vi "destroySubDataUserEvents.vi"(8 "error in (no error)":errorcluster, 11 "PubSubDataEvent in":refnum<class "PubSubDataEvent.lvclass">) -> (0 "error out":errorcluster, 3 "PubSubDataEvent out":refnum<class "PubSubDataEvent.lvclass">)   [LabVIEW 2016, in "PubSubDataEvent.lvclass"]
uses:
  PubSubDataEvent.lvclass
  PubSubDataEvent.lvclass/PubSubDataEvent.ctl
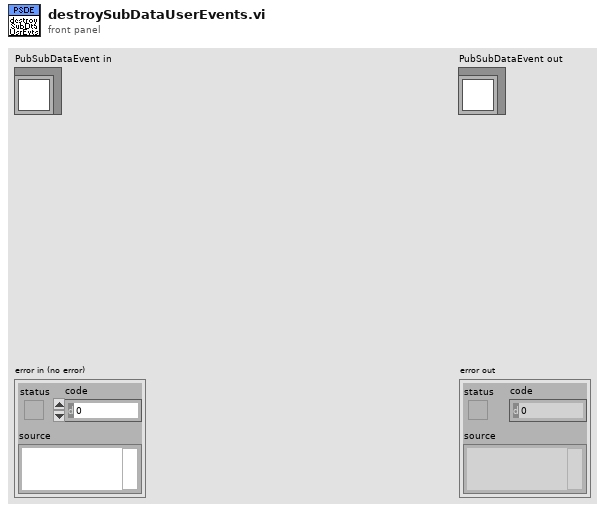
[diagram p1: front panel]
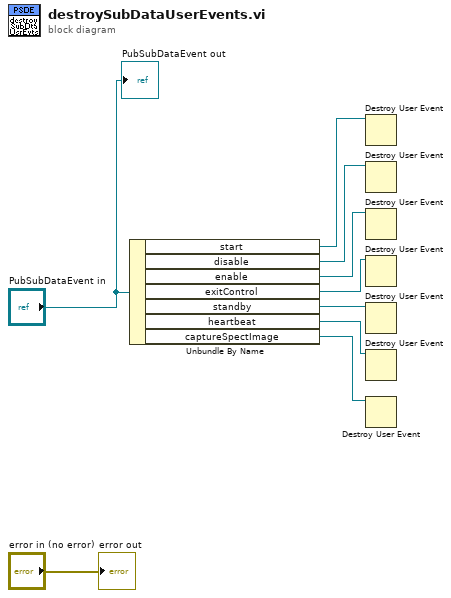
[diagram p0: block diagram]
diagram:
  n1 = Unbundle By Name("PubSubDataEvent in") -> ("start"=w7:refnum<user-event>, "disable"=w6:refnum<user-event>, "enable"=w5:refnum<user-event>, "exitControl"=w4:refnum<user-event>, "standby"=w3:refnum<user-event>, "heartbeat"=w2:refnum<user-event>, "captureSpectImage"=w1:refnum<user-event>)
  n2 = Destroy User Event(user event=w7) -> ()  [unwired: 1 in, 1 out]
  n3 = Destroy User Event(user event=w6) -> ()  [unwired: 1 in, 1 out]
  n4 = Destroy User Event(user event=w5) -> ()  [unwired: 1 in, 1 out]
  n5 = Destroy User Event(user event=w4) -> ()  [unwired: 1 in, 1 out]
  n6 = Destroy User Event(user event=w3) -> ()  [unwired: 1 in, 1 out]
  n7 = Destroy User Event(user event=w2) -> ()  [unwired: 1 in, 1 out]
  n8 = Destroy User Event(user event=w1) -> ()  [unwired: 1 in, 1 out]
  "error out" <- "error in (no error)"
  "PubSubDataEvent out" <- "PubSubDataEvent in"
